vi "fn Status.vi"(8 "error in (no error)":errorcluster, 11 "LV_status":string) -> (0 "error out":errorcluster, 2 "function return":i32, 3 "LV_status out":string)   [LabVIEW 2018, in "LV_OPC.lvlib"]
doc: "LVOPC_API int fnStatus(char* LV_status);"
uses:
  LV_OPC.lvlib
  LVOPC64.dll
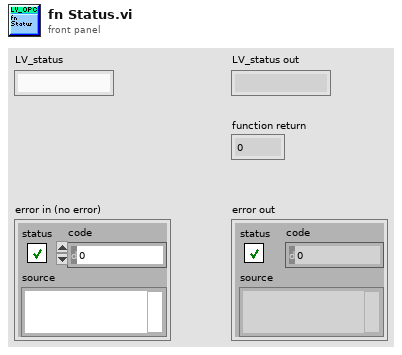
[diagram p1: front panel]
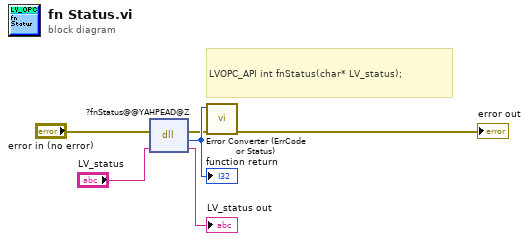
[diagram p0: block diagram]
diagram:
  # "LVOPC_API int fnStatus(char* LV_status);"
  n1 = dll-call lib="C:/Users/Andrey/Desktop/LV_OPC-Client-x64/LV_OPC_Test/OPC.DLL/LVOPC64.*" fn="?fnStatus@@YAHPEAD@Z"(error in="error in (no error)", "LV_status"="LV_status") -> (error out=w2:errorcluster, "return type"=w6:i32, "LV_status"=→"LV_status out":string)  [unwired: 2 in, 1 out]
  "function return" <- w6
  n2 = call "Error Converter (ErrCode or Status).vi"("error in (no error)"=w2, "error code"=w6) -> ("error out"=→"error out":errorcluster)  [unwired: 9 in]
